vi "OpenClaw.vi"(8 "error in":errorcluster, 9 "FPGA VI Reference In":T1, 10 "milliseconds to wait \nfor servo to change":u32=100, 11 "Old Angle":dbl) -> (0 "error out":errorcluster, 1 "FPGA VI Reference Out":T1, 2 "milliseconds to wait \nfor servo to change Out":u32, 3 "New Angle":dbl)   [LabVIEW 2012]
uses:
  FPGA_ref.ctl
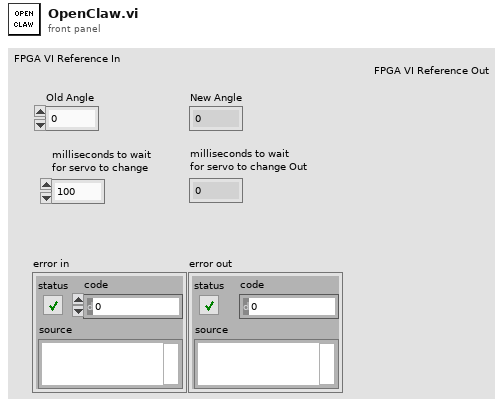
[diagram p1: front panel]
types:
  T1 = typedef "FPGA_ref.ctl" = refnum<k20>
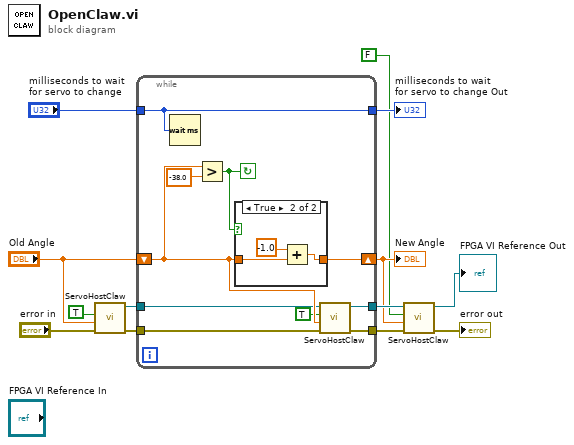
[diagram p0: block diagram]
diagram:
  n1 = call "ServoHostClaw.vi"("error in"="error in", "Angle (deg) Claw"="Old Angle", "Enable"=TRUE) -> ("error out"=w10:errorcluster, "FPGA VI Reference Out"=w11:T1)  [unwired: 7 in]
  n2 = while {
    tunnel: w10 -> [w19]
    shift-right: [w22] -> w2
    shift-left: "Old Angle" -> [w18]
    tunnel: "milliseconds to wait \nfor servo to change" -> [w20]
    tunnel: [w17] -> w4
    tunnel: [w20] -> w12
    tunnel: w11 -> [w16]
    tunnel: [w15] -> w7
    stop <- w21 continue-if-true
    n3 = Wait (ms)(milliseconds to wait=w20) -> ()  [unwired: 1 out]
    n4 = Greater?(x=w18, y=-38.0) -> (0:w21:bool)
    n5 = case shown="True" w21 {
      tunnel: [w24 w26] -> w22
      tunnel: w18 -> [w24 w25]
      frame False {
      }
      frame True {
        n6 = Add(x=-1.0, y=w25) -> (x+y=w26:dbl)
      }
    }
    n7 = call "ServoHostClaw.vi"("error in"=w19, "Angle (deg) Claw"=w18, "Enable"=TRUE, "FPGA VI Reference In"=w16) -> ("error out"=w17:errorcluster, "FPGA VI Reference Out"=w15:T1)  [unwired: 6 in]
  }
  "New Angle" <- w2
  "milliseconds to wait \nfor servo to change Out" <- w12
  n8 = call "ServoHostClaw.vi"("error in"=w4, "Angle (deg) Claw"=w2, "Enable"=FALSE, "FPGA VI Reference In"=w7) -> ("error out"=→"error out":errorcluster, "FPGA VI Reference Out"=→"FPGA VI Reference Out":T1)  [unwired: 6 in]
